vi "ReadExecution Count.vi"(8 "error in (no error)":errorcluster, 11 "object in":refnum<class "execute_result Message.lvclass">) -> (0 "error out":errorcluster, 2 "Execution Count":i32, 3 "object out":refnum<class "execute_result Message.lvclass">)   [LabVIEW 2018, in "ClientMessaging.lvlib" / "execute_result Message.lvclass"]
uses:
  execute_result Message.lvclass
  execute_result Message.lvclass/execute_result Message.ctl
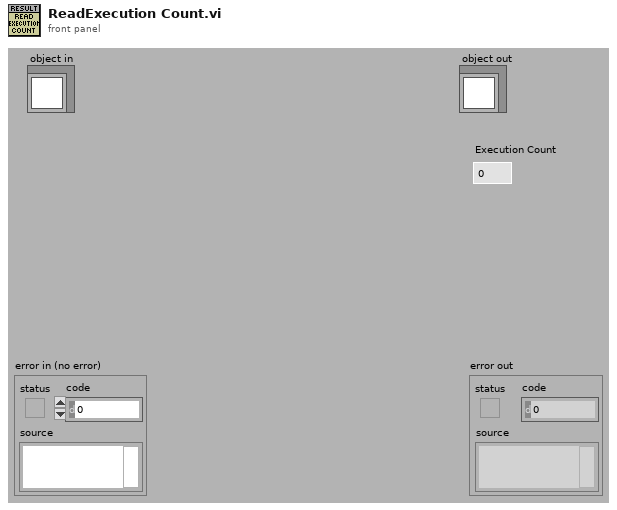
[diagram p1: front panel]
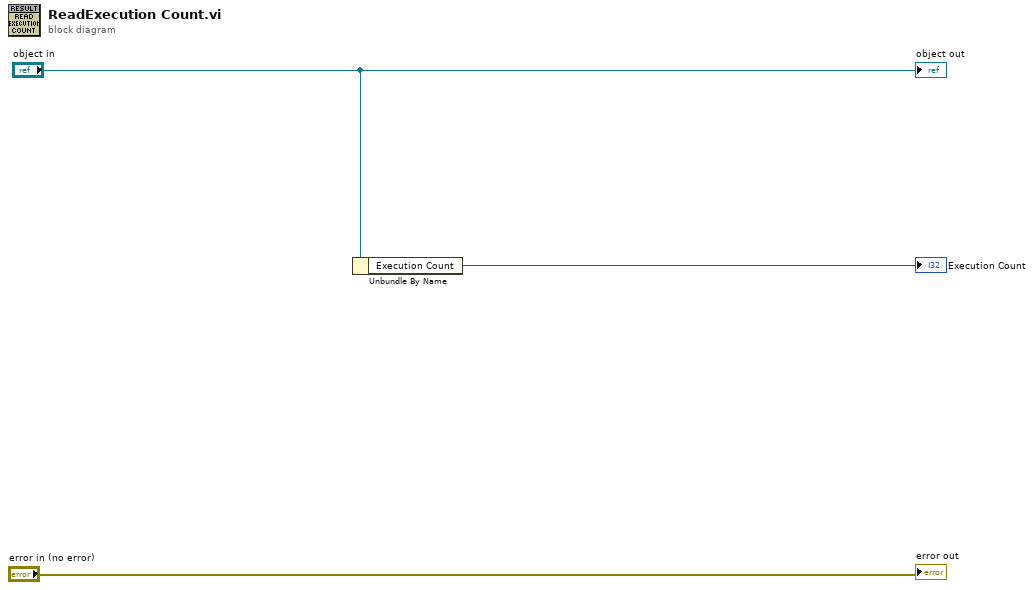
[diagram p0: block diagram]
diagram:
  n1 = Unbundle By Name("object in") -> ("Execution Count"=→"Execution Count":i32)
  "error out" <- "error in (no error)"
  "object out" <- "object in"
